vi "UDP_Client_Producer_Consumer.vi"() -> ()   [LabVIEW 2021]
panel:
  out "Dequeue loop specific error cleared":bool
  out "Enque loop specific error cleared":bool
  out "release queque specific error cleared":bool
  out "Enqueued Data":dbl[](array[numeric])
  out "Transmitted data":waveform(dbl)(graph)
  out "Dequed Data":waveform(dbl)(graph)
  out "Dequed Data":dbl[](array[numeric])
  out "Transmitted data":dbl[](array[numeric])
  out "Enqueued Data":waveform(dbl)(graph)
  out "Dequeque monitor":dbl(graph)
  in  "stop":bool
  out "error out":errorcluster
  in  "A(t)":dbl(knob) min=0.0 max=1.0 scale=0.0..1.0
  # "Enqueued Data"
  # "Dequeued Data"
  # "Transmitted Data"
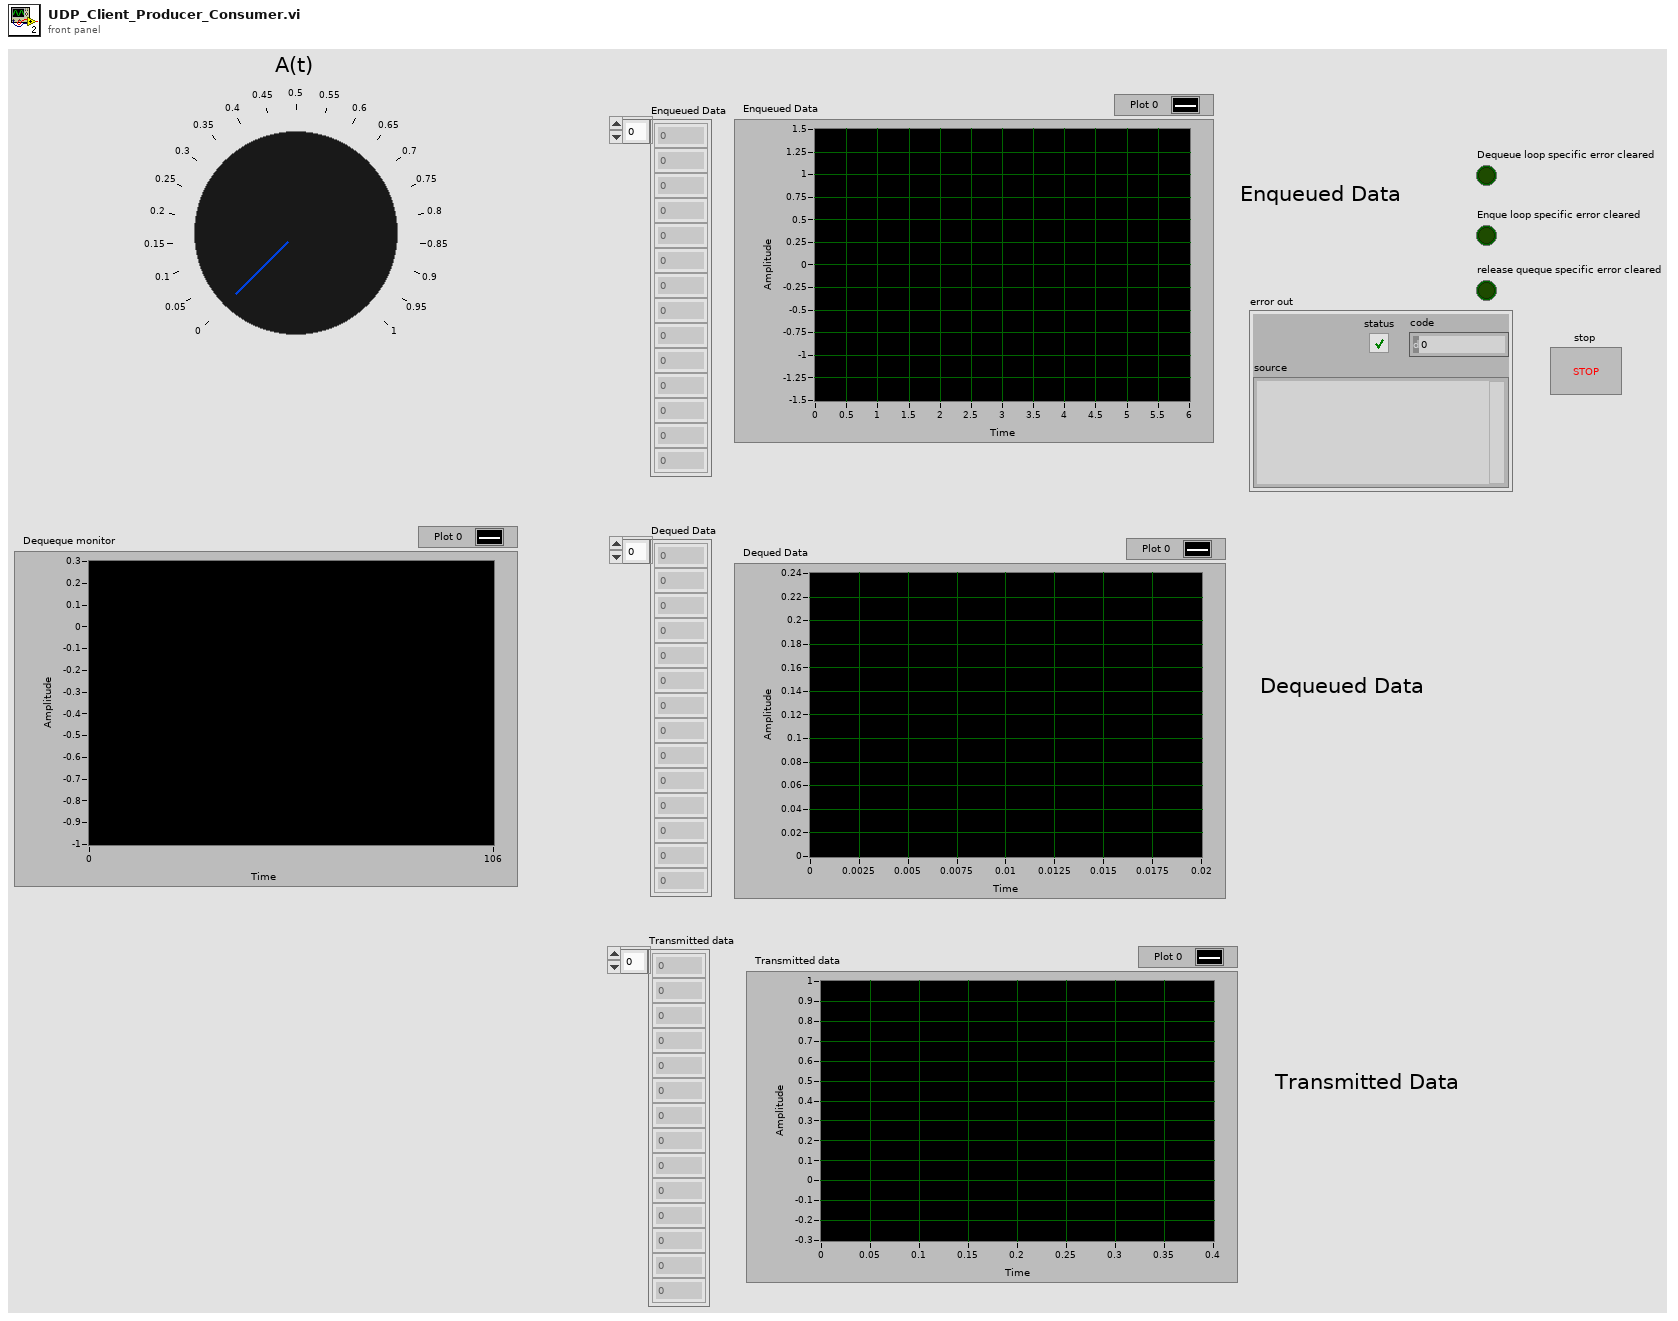
[diagram p1: front panel]
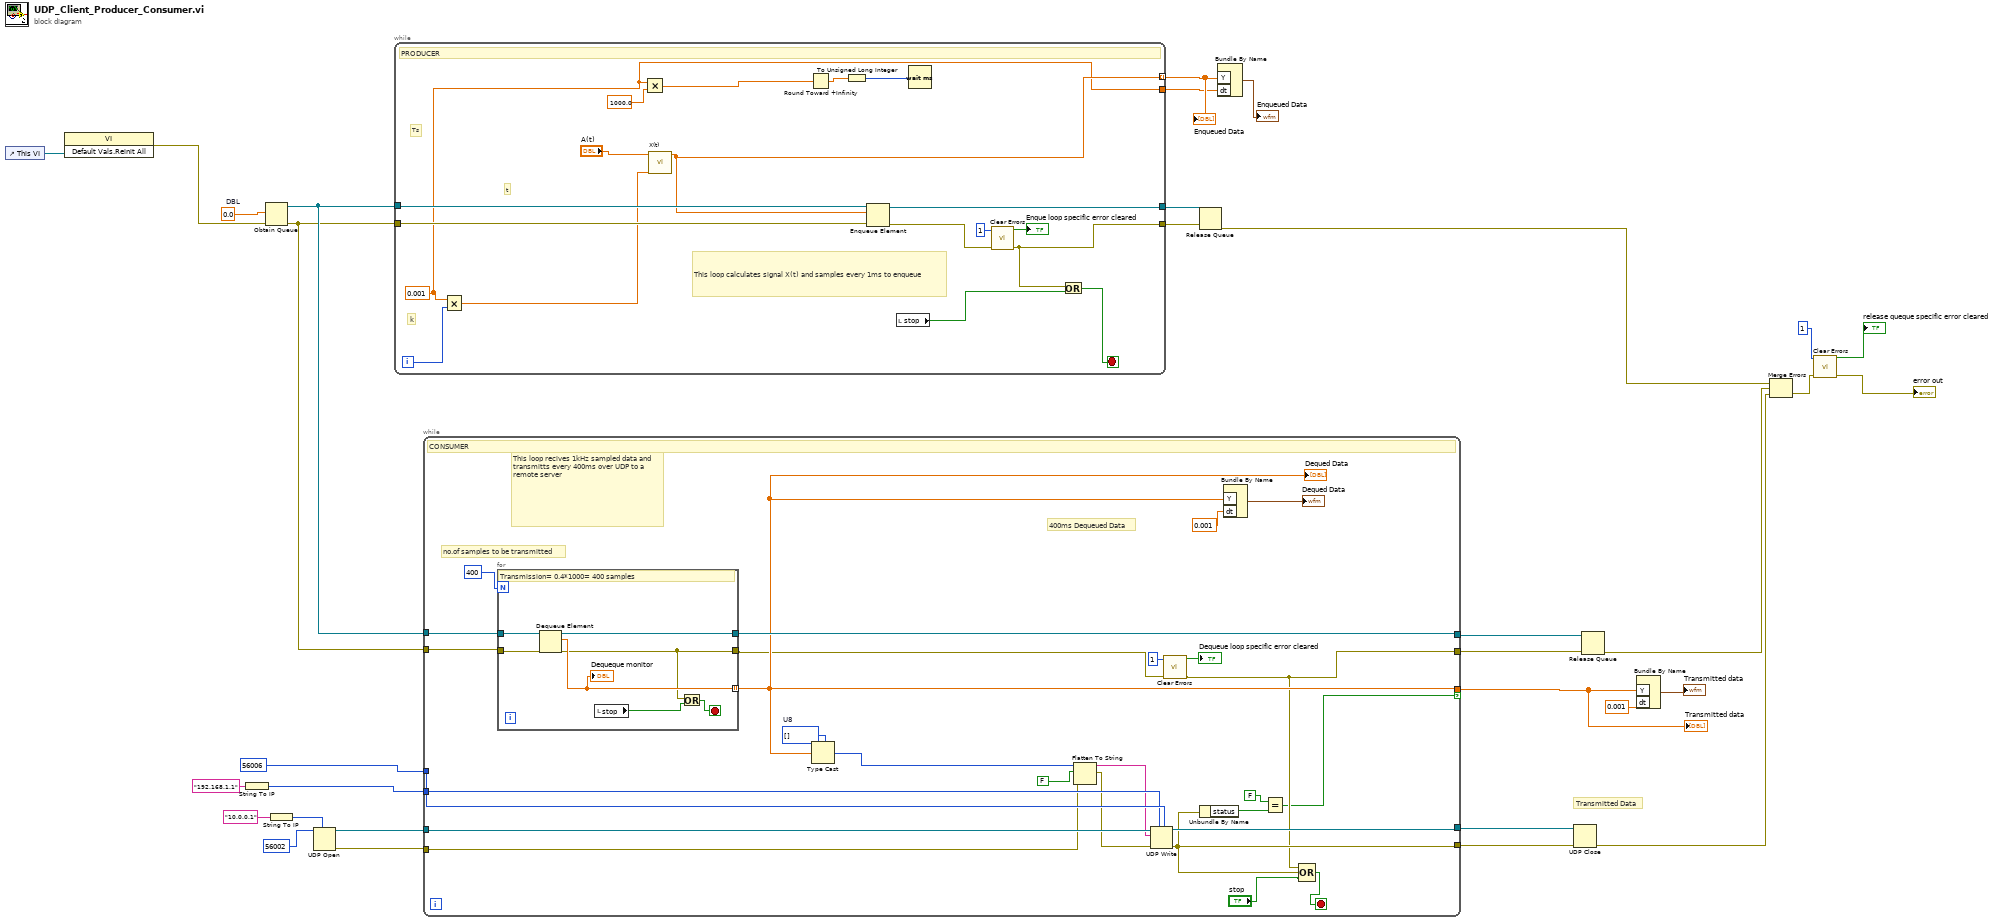
[diagram p0: block diagram]
diagram:
  w32 = 0.0  # DBL
  # "Transmitted Data"
  n1 = control-ref of="This VI"() -> (w12:refnum<vi>)
  n2 = invoke class="VI" method="Default Vals.Reinit All"(reference=w12) -> (error out=w5:errorcluster)  [unwired: 2 in, 2 out]
  n3 = String To IP(1:"192.168.1.1" ("name")) -> (0:w13:u32)
  n4 = Obtain Queue(element data type=w32, error in (no error)=w5) -> (queue out=w25:refnum<queue>, error out=w23:errorcluster)  [unwired: 3 in, 1 out]
  n5 = String To IP(1:"10.0.0.1" ("name")) -> (0:w17:u32)
  n6 = UDP Open(7:w17, 11:u16 56002 ("port")) -> (port=w29:refnum<k16>, 0:w27:errorcluster)  [unwired: 3 in, 1 out]
  n7 = while {
    tunnel: w25 -> [w50]
    tunnel: w23 -> [w49]
    tunnel: [w48] -> w31
    tunnel: [w33] -> w30
    tunnel: [w40] -> w10 mode=indexing
    tunnel: [w39] -> w9
    i -> [w47]
    stop <- w37 stop-if-true
    w39 = 0.001
    # "This loop calculates signal X(t) and samples every 1ms to enqueue"
    # "t"
    # "k"
    # "Ts"
    # "PRODUCER"
    n8 = Multiply(x=w39, y=w47) -> (x*y=w41:dbl)
    n9 = Multiply(x=w39, y=1000.0) -> (x*y=w42:dbl)
    n10 = call "X(t).vi"("t"=w41, "A(t)"="A(t)") -> ("X(t)"=w40:dbl)  [unwired: 9 in]
    n11 = Round Toward +Infinity(x=w42) -> (ceil(x): smallest int >= x=w45:dbl)
    n12 = To Unsigned Long Integer(number=w45) -> (unsigned 32bit integer=w44:u32)
    n13 = Enqueue Element(queue=w50, element=w40, error in (no error)=w49) -> (queue out=w48:refnum<queue>, error out=w34:errorcluster)  [unwired: 1 in, 1 out]
    n14 = local read "stop"() -> (w38:bool)
    n15 = Wait (ms)(milliseconds to wait=w44) -> ()  [unwired: 1 out]
    n16 = call <vilib>:"Clear Errors.vi"("error in (no error)"=w34, "specific error code to clear (0: all)"=1) -> ("error out"=w33:errorcluster, "specific error cleared?"=→"Enque loop specific error cleared":bool)  [unwired: 4 in]
    n17 = Or(x=w33, y=w38) -> (x .or. y?=w37:bool)
  }
  "Enqueued Data" <- w10
  n18 = while {
    tunnel: w29 -> [w77]
    tunnel: [w76] -> w28
    tunnel: w27 -> [w60]
    tunnel: [w58] -> w26
    tunnel: w25 -> [w75]
    tunnel: [w74] -> w24
    tunnel: w23 -> [w73]
    tunnel: [w52] -> w22
    tunnel: u16 56006 ("port") -> [w72]
    tunnel: w13 -> [w71]
    tunnel: [w61] -> w6 if=w51
    stop <- w56 stop-if-true
    w70 = u8[] []  # U8
    # "no.of samples to be transmitted"
    # "This loop recives 1kHz sampled data and transmitts every 400ms over UDP to a remote server"
    # "400ms Dequeued Data"
    # "CONSUMER"
    n19 = for {
      N: 400 -> [_]
      tunnel: w75 -> [w84]
      tunnel: [w83] -> w74
      tunnel: w73 -> [w82]
      tunnel: [w79] -> w53
      tunnel: [w81] -> w61 mode=indexing
      stop <- w78 stop-if-true
      # "Transmission= 0.4*1000= 400 samples"
      n20 = Dequeue Element(queue=w84, error in (no error)=w82) -> (queue out=w83:refnum<queue>, element=w81:dbl, error out=w79:errorcluster)  [unwired: 1 in, 1 out]
      "Dequeque monitor" <- w81
      n21 = local read "stop"() -> (w80:bool)
      n22 = Or(x=w79, y=w80) -> (x .or. y?=w78:bool)
    }
    "Dequed Data" <- w61
    n23 = Type Cast(type=w70, x=w61) -> (*(type *) &x=w68:u8[])
    n24 = Flatten To String(anything=w68, prepend array or string size? (T)=FALSE, error in (no error)=w60) -> (data string=w66:string, error out=w59:errorcluster)  [unwired: 1 in, 1 out]
    n25 = UDP Write(address=w71, port or service name=w72, connection ID=w77, data in=w66, 8:w59) -> (error out=w58:errorcluster, 3:w76:refnum<k16>)  [unwired: 1 in]
    n26 = call <vilib>:"Clear Errors.vi"("error in (no error)"=w53, "specific error code to clear (0: all)"=1) -> ("error out"=w52:errorcluster, "specific error cleared?"=→"Dequeue loop specific error cleared":bool)  [unwired: 4 in]
    n27 = Unbundle By Name(w58) -> ("status"=w65:bool)
    n28 = Bundle By Name("Y"=w61, "dt"=0.001) -> (→"Dequed Data":waveform(dbl))  [unwired: 1 in]
    n29 = Equal?(x=FALSE, y=w65) -> (x = y?=w51:bool)
    n30 = Compound Arithmetic op=OR(w52, w58, "stop") -> (w56:bool)
  }
  "Transmitted data" <- w6
  n31 = Release Queue(queue=w31, error in (no error)=w30) -> (error out=w21:errorcluster)  [unwired: 1 in, 2 out]
  n32 = Bundle By Name("Y"=w10, "dt"=w9) -> (→"Enqueued Data":waveform(dbl))  [unwired: 1 in]
  n33 = UDP Close(connection ID=w28, 8:w26) -> (error out=w19:errorcluster)  [unwired: 1 out]
  n34 = Release Queue(queue=w24, error in (no error)=w22) -> (error out=w20:errorcluster)  [unwired: 1 in, 2 out]
  n35 = Bundle By Name("Y"=w6, "dt"=0.001) -> (→"Transmitted data":waveform(dbl))  [unwired: 1 in]
  n36 = Merge Errors(w21, w20, w19) -> (w4:errorcluster)
  n37 = call <vilib>:"Clear Errors.vi"("error in (no error)"=w4, "specific error code to clear (0: all)"=1) -> ("error out"=→"error out":errorcluster, "specific error cleared?"=→"release queque specific error cleared":bool)  [unwired: 4 in]
